vi "Param Class.vi"(11 "Promise in":refnum<class "Promise.lvclass">) -> (2 "Param Class":string)   [LabVIEW 2020, in "Promises.lvlib" / "Promise.lvclass"]
uses:
  Promise.lvclass
  Promise.lvclass/Promise.ctl
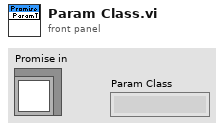
[diagram p1: front panel]
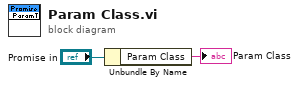
[diagram p0: block diagram]
diagram:
  n1 = Unbundle By Name("Promise in") -> ("Param Class"=→"Param Class":string)
